vi "Write Ctl Refnum.vi"(8 "error in (no error)":errorcluster, 10 "Ctl Refnum":refnum<vi>, 11 "Button in":refnum<class "Button.lvclass">) -> (0 "error out":errorcluster, 3 "Button out":refnum<class "Button.lvclass">)   [LabVIEW 2020, in "Button.lvclass"]
uses:
  Button.lvclass
  Button.lvclass/Button.ctl
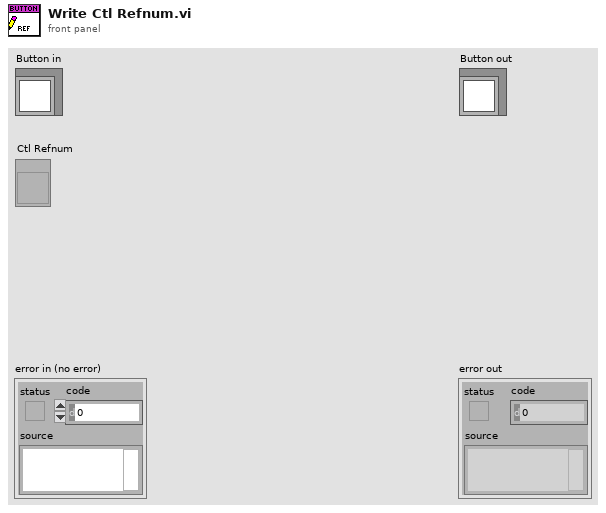
[diagram p1: front panel]
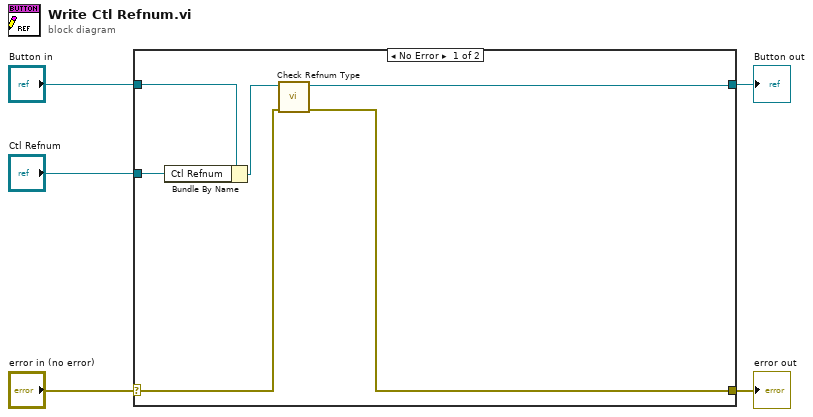
[diagram p0: block diagram]
diagram:
  n1 = case shown="No Error" "error in (no error)" {
    selector: "error in (no error)" -> [w8 w12]
    tunnel: [w6 w12] -> w4
    tunnel: [w7 w13] -> w2
    tunnel: "Button in" -> [w11 w13]
    tunnel: "Ctl Refnum" -> [w10 _]
    frame No Error {
      n2 = Bundle By Name(cluster=w11, "Ctl Refnum"=w10) -> (w9:refnum<class "Button.lvclass">)
      n3 = call-dynamic "Check Refnum Type.vi"("error in (no error)"=w8, "Button in"=w9) -> ("error out"=w6:errorcluster, "Button out"=w7:refnum<class "Button.lvclass">)  [unwired: 8 in]
    }
    frame Error {
    }
  }
  "error out" <- w4
  "Button out" <- w2
